vi "S8300E_SetRTCTime_FromSFCS.vi"() -> ()   [LabVIEW 2011]
uses:
  Instance           3 34Saved   MojoMP_SetRTCTime_FromSFCS .vi
  Instance           5 34Saved   MojoMP_SetRTCTime_FromSFCS .vi
  Instance           6 34Saved   MojoMP_SetRTCTime_FromSFCS .vi
  data/MCSDLL.dll
panel:
  out "UUT Msg":string
  out "SFCS Msg":string
  out "VISA resource name out":refnum<visa-resource-name>
  out "begin time":u32
  out "toS8300E_RTC_Data":string
  out "SFCS_Time":string
  out "SFCS_DATE_STRING":string
  out "output param":string
  out "STAGE":string
  out "SFCS_IP":string
  in  "URL":string
  # "設定標準時間\nSetRTC Time from SFCS To S8300E"
  # "2014-9-3"
  # "Error Code:RTC\nError Code:UART"
  # "COM9"
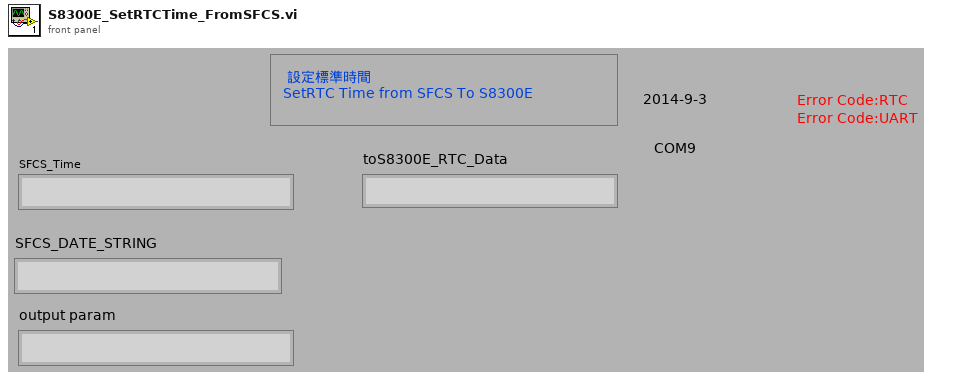
[diagram p1: front panel]
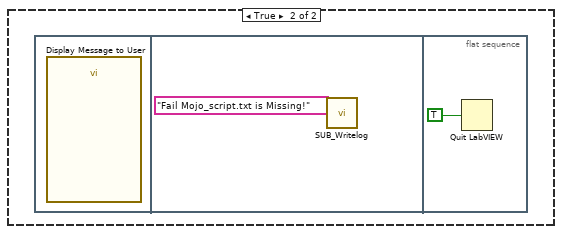
[diagram p3: hidden frame]
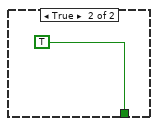
[diagram p9: hidden frame]
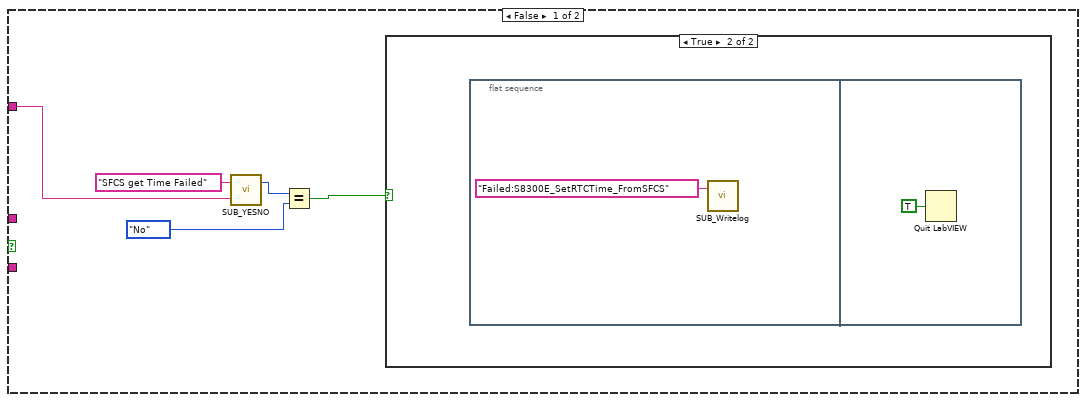
[diagram p10: hidden frame]
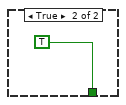
[diagram p13: hidden frame]
diagram:
  n1 = flat-sequence {
    tunnel: [w4] -> w1
    tunnel: w1 -> [w27]
    frame #0 {
      n2 = Tick Count (ms)() -> (millisecond timer value=→"begin time":u32)
    }
    frame #1 {
      n3 = call "SUB_Read_specifFile.vi"("name or relative path"="S8300E_sfcs_misc.txt" ("Script FileName")) -> ("error out"=w7:errorcluster, "text"=w4:string)  [unwired: 1 in]
      n4 = Unbundle By Name(w7) -> ("code"=w6:i32)
      n5 = Not Equal To 0?(x=w6) -> (x != 0?=w5:bool)
      n6 = case shown="False" w5 {
        tunnel: w4 -> [w8 _]
        frame False {
          n7 = flat-sequence {
            tunnel: w8 -> [w14]
            frame #0 {
              n8 = To Upper Case(1:"SFCS_IP=" ("string")) -> (0:w18:string)
              n9 = To Upper Case(1:w14) -> (0:w19:string)
              n10 = call <vilib>:"Trim Whitespace.vi"("string"=w18) -> ("trimmed string"=w16:string)  [unwired: 1 in]
              n11 = call <vilib>:"Trim Whitespace.vi"("string"=w19) -> ("trimmed string"=w15:string)  [unwired: 1 in]
              n12 = Match Pattern(string=w15, regular expression=w16) -> (after substring=w13:string)  [unwired: 1 in, 3 out]
              n13 = Match Pattern(string=w13, regular expression=";") -> (before substring=w11:string)  [unwired: 1 in, 3 out]
              "SFCS_IP" <- w11
              n14 = Equal?(x=w11, y="") -> (x = y?=w9:bool)
              n15 = case shown="True" w9 {
                frame False {
                }
                frame True {
                  n16 = flat-sequence {
                    frame #0 {
                      n17 = call "Display Message to User2"() -> ()  [unwired: 10 in, 2 out]
                    }
                    frame #1 {
                      n18 = call "SUB_Writelog.vi"("Pass/Fail"="Fail Not Found SFCS_IP=\"xx.xx.xx.xx\" in Mojo_script.txt !") -> ()  [unwired: 2 in]
                    }
                    frame #2 {
                      n19 = Quit LabVIEW(quit? (T)=TRUE) -> ()
                    }
                  }
                }
              }
            }
          }
        }
        frame True {
          n20 = flat-sequence {
            frame #0 {
              n21 = call "Display Message to User"() -> ()  [unwired: 10 in, 2 out]
            }
            frame #1 {
              n22 = call "SUB_Writelog.vi"("Pass/Fail"="Fail Mojo_script.txt is Missing!") -> ()  [unwired: 2 in]
            }
            frame #2 {
              n23 = Quit LabVIEW(quit? (T)=TRUE) -> ()
            }
          }
        }
      }
    }
    frame #2 {
      n24 = To Upper Case(1:"SFCS_STAGE=" ("string")) -> (0:w33:string)
      n25 = To Upper Case(1:w27) -> (0:w34:string)
      n26 = call <vilib>:"Trim Whitespace.vi"("string"=w33) -> ("trimmed string"=w32:string)  [unwired: 1 in]
      n27 = call <vilib>:"Trim Whitespace.vi"("string"=w34) -> ("trimmed string"=w31:string)  [unwired: 1 in]
      n28 = Match Pattern(string=w31, regular expression=w32) -> (after substring=w30:string)  [unwired: 1 in, 3 out]
      n29 = Match Pattern(string=w30, regular expression=";") -> (before substring=w26:string)  [unwired: 1 in, 3 out]
      "STAGE" <- w26
      n30 = Not Equal?(x=w26, y="") -> (x != y?=w24:bool)
      n31 = case shown="False" w24 {
        frame False {
          n32 = flat-sequence {
            frame #0 {
              n33 = call "Display Message to User4"() -> ()  [unwired: 10 in, 2 out]
            }
            frame #1 {
              n34 = call "SUB_Writelog.vi"("Pass/Fail"="Fail :Stage  not define in script file!") -> ()  [unwired: 2 in]
            }
            frame #2 {
              n35 = Quit LabVIEW(quit? (T)=TRUE) -> ()
            }
          }
        }
        frame True {
        }
      }
    }
    frame #3 {
      n36 = local read "SFCS_IP"() -> (w37:string)
      n37 = local write "URL"(w37) -> ()
    }
    frame #4 {
      n38 = case shown="True" TRUE {
        frame False {
        }
        frame True {
          n39 = call "SUB_COM1_CLOSE.vi"("VISA resource name"=refnum<visa-resource-name> "COM9") -> ()  [unwired: 3 in]
        }
      }
    }
    frame #5 {
      n40 = case shown="True" TRUE {
        frame False {
        }
        frame True {
          n41 = call "SUB_COM9_INIT.vi"("baud rate"=u32 115200) -> ("VISA resource name out"=w44:refnum<visa-resource-name>)  [unwired: 1 in, 1 out]
          "VISA resource name out" <- w44
          n42 = call "SUB_COM1Wrt.vi"("VISA resource name"=w44, "write buffer"="\r") -> ("duplicate VISA resource name"=w41:refnum<visa-resource-name>)  [unwired: 2 out]
          n43 = call "SUB_ContinueCom1Read.vi"("Numeric"=1200, "duplicate VISA resource name 2"=w41) -> ()  [unwired: 1 in, 3 out]
        }
      }
    }
    frame #6 {
      n44 = case shown="True" TRUE {
        frame False {
        }
        frame True {
          n45 = while {
            stop <- w56 stop-if-true
            w49 = "S8300E" ("Find this String")
            w50 = "\r"
            n46 = Tick Count (ms)() -> (millisecond timer value=w53:u32)
            n47 = local read "VISA resource name out"() -> (w55:refnum<visa-resource-name>)
            n48 = Concatenate Strings(w50, w50, w50) -> (w51:string)
            n49 = call "SUB_COM1Wrt.vi"("VISA resource name"=w55, "write buffer"=w51) -> ("duplicate VISA resource name"=w54:refnum<visa-resource-name>)  [unwired: 2 out]
            n50 = call "SUB_READ_COM1_FindString_timeout.vi"("Find this String"=w49, "Timeout Seccond"=3.0, "Begin time"=w53, "duplicate VISA resource name 2"=w54) -> ("Output String"=w48:string)  [unwired: 1 in, 2 out]
            n51 = call "SUB_FindSpecificString.vi"("Find this String"=w49, "String data"=w48) -> ("Found"=w47:bool)  [unwired: 2 in, 1 out]
            n52 = case shown="False" w47 {
              tunnel: w48 -> [w61 _]
              tunnel: [w57 TRUE] -> w56
              frame False {
                n53 = call "SUB_YESNO.vi"("Debug View"=w61, "Status"="UART無正確反應!需有S8300E字串") -> ("yes/no"=w60:enum32{"No Selection", "Yes", "No", "None"})  [unwired: 1 in]
                n54 = Equal?(x=w60, y=enum32{"No Selection", "Yes", "No", "None"}."No") -> (x = y?=w58:bool)
                n55 = case shown="True" w58 {
                  tunnel: [_ w63] -> w57
                  frame False {
                  }
                  frame True {
                    n56 = flat-sequence {
                      tunnel: [w67] -> w63
                      frame #0 {
                        n57 = call "SUB_Writelog.vi"("Pass/Fail"="Fail:S8300E_SetRTCTime_FromSFCS") -> ()  [unwired: 2 in]
                      }
                      frame #1 {
                        n58 = call "SUB_SFCS_SendResult.vi"("ErrorCode"="UART", "PASS_Fail (1/0)"=i8 0) -> ()  [unwired: 1 out]
                      }
                      frame #2 {
                        w67 = TRUE ("quit? (T)")
                        n59 = Quit LabVIEW(quit? (T)=w67) -> ()
                      }
                    }
                  }
                }
              }
              frame True {
              }
            }
          }
        }
      }
    }
    frame #7 {
      n60 = while {
        stop <- w69 stop-if-true
        w86 = ":" ("regular expression")
        w88 = "/" ("regular expression")
        w90 = " " ("regular expression")
        n61 = local read "STAGE"() -> (w94:string)
        n62 = To Upper Case(1:"NG" ("string")) -> (0:w101:string)
        n63 = To Upper Case(1:"Fail" ("string")) -> (0:w78:string)
        n64 = call <vilib>:"Trim Whitespace.vi"("string"=w101) -> ("trimmed string"=w98:string)  [unwired: 1 in]
        n65 = call <vilib>:"Trim Whitespace.vi"("string"=w78) -> ("trimmed string"=w75:string)  [unwired: 1 in]
        n66 = dll-call lib="D:/S8300E_Project/data/MCSDLL.dll" fn="SFCS_GetCurrentDBSysdate"("URL"="URL", "Stage"=w94, "TimeFormat"="YYYY/MM/DD HH24:MI:SS") -> (w70:string)  [unwired: 6 in, 2 out]
        "output param" <- w70
        "SFCS Msg" <- w70
        n67 = To Upper Case(1:w70) -> (0:w102:string)
        n68 = To Upper Case(1:w70) -> (0:w79:string)
        n69 = call <vilib>:"Trim Whitespace.vi"("string"=w102) -> ("trimmed string"=w97:string)  [unwired: 1 in]
        n70 = call <vilib>:"Trim Whitespace.vi"("string"=w79) -> ("trimmed string"=w74:string)  [unwired: 1 in]
        n71 = Match Pattern(string=w97, regular expression=w98) -> (match substring=w99:string)  [unwired: 1 in, 3 out]
        n72 = Match Pattern(string=w74, regular expression=w75) -> (match substring=w76:string)  [unwired: 1 in, 3 out]
        n73 = Not Equal?(x=w99, y=w98) -> (x != y?=w73:bool)
        n74 = Not Equal?(x=w76, y=w75) -> (x != y?=w72:bool)
        n75 = Match Pattern(string=w70, regular expression=w86) -> (match substring=w87:string)  [unwired: 1 in, 3 out]
        n76 = Match Pattern(string=w70, regular expression=w88) -> (match substring=w89:string)  [unwired: 1 in, 3 out]
        n77 = And(x=w73, y=w72) -> (x .and. y?=w71:bool)
        n78 = Equal?(x=w89, y=w88) -> (x = y?=w83:bool)
        n79 = Equal?(x=w87, y=w86) -> (x = y?=w85:bool)
        n80 = Match Pattern(string=w70, regular expression=w90) -> (before substring=w93:string, match substring=w91:string, after substring=w92:string)  [unwired: 1 in, 1 out]
        n81 = And(x=w85, y=w71) -> (x .and. y?=w81:bool)
        n82 = Equal?(x=w91, y=w90) -> (x = y?=w84:bool)
        n83 = And(x=w84, y=w83) -> (x .and. y?=w82:bool)
        n84 = And(x=w82, y=w81) -> (x .and. y?=w80:bool)
        n85 = case shown="True" w80 {
          tunnel: w93 -> [_ w115]
          tunnel: w92 -> [_ w114]
          tunnel: w70 -> [w103 _]
          tunnel: [_ w113] -> w69
          frame False {
            n86 = call "SUB_YESNO.vi"("Debug View"=w103, "Status"="SFCS get Time Failed") -> ("yes/no"=w106:enum32{"No Selection", "Yes", "No", "None"})  [unwired: 1 in]
            n87 = Equal?(x=w106, y=enum32{"No Selection", "Yes", "No", "None"}."No") -> (x = y?=w104:bool)
            n88 = case shown="True" w104 {
              frame False {
              }
              frame True {
                n89 = flat-sequence {
                  frame #0 {
                    n90 = call "SUB_Writelog.vi"("Pass/Fail"="Failed:S8300E_SetRTCTime_FromSFCS") -> ()  [unwired: 2 in]
                  }
                  frame #1 {
                    n91 = Quit LabVIEW(quit? (T)=TRUE) -> ()
                  }
                }
              }
            }
          }
          frame True {
            n92 = flat-sequence {
              tunnel: w115 -> [w131]
              tunnel: w114 -> [w130]
              tunnel: [w117] -> w112
              tunnel: w112 -> [w133]
              tunnel: [w132] -> w110
              tunnel: [w137] -> w111
              tunnel: w110 -> [w137]
              tunnel: [w145] -> w113
              tunnel: w111 -> [w139]
              frame #0 {
                n93 = call <vilib>:"Trim Whitespace.vi"("string"=w131) -> ("trimmed string"=w122:string)  [unwired: 1 in]
                "SFCS_DATE_STRING" <- w122
                n94 = call <vilib>:"Trim Whitespace.vi"("string"=w130) -> ("trimmed string"=w129:string)  [unwired: 1 in]
                "SFCS_Time" <- w129
                n95 = call "SUB_OUT_THIS_token.vi"("Remove token symbl1 3"="", "Remove token symbl1 2"=":" ("Remove token symbl1"), "Remove token symbl1"="/", "input string"=w129) -> ("result string"=w120:string)  [unwired: 1 in]
                n96 = call "SUB_OUT_THIS_token.vi"("Remove token symbl1 3"="", "Remove token symbl1 2"=":" ("Remove token symbl1"), "Remove token symbl1"="/", "input string"=w122) -> ("result string"=w121:string)  [unwired: 1 in]
                n97 = Concatenate Strings(w121, w120) -> (w116:string)
                "toS8300E_RTC_Data" <- w116
                n98 = Concatenate Strings("./rtc.sh -w  ", w116, "\r") -> (w117:string)
              }
              frame #1 {
                n99 = local read "VISA resource name out"() -> (w135:refnum<visa-resource-name>)
                n100 = call "SUB_ContinueCom1Read.vi"("Numeric"=1200, "duplicate VISA resource name 2"=w135) -> ("duplicate VISA resource name"=w134:refnum<visa-resource-name>)  [unwired: 1 in, 2 out]
                n101 = call "SUB_COM1Wrt.vi"("VISA resource name"=w134, "write buffer"=w133) -> ("duplicate VISA resource name"=w132:refnum<visa-resource-name>)  [unwired: 2 out]
              }
              frame #2 {
                n102 = Wait (ms)(milliseconds to wait=u32 3000) -> ()  [unwired: 1 out]
              }
              frame #3 {
                n103 = Tick Count (ms)() -> (millisecond timer value=w141:u32)
                n104 = call "SUB_READ_COM1_FindString_timeout.vi"("Find this String"="PASSED=", "Timeout Seccond"=1.0, "Begin time"=w141, "duplicate VISA resource name 2"=w139) -> ("Output String"=→"UUT Msg":string, "Found String"=w143:bool)  [unwired: 1 in, 1 out]
                n105 = case shown="False" w143 {
                  tunnel: [_ TRUE] -> w145
                  frame False {
                    n106 = local read "UUT Msg"() -> (w149:string)
                    n107 = call "SUB_YESNO.vi"("Debug View"=w149, "Status"="設定RTC失敗!") -> ("yes/no"=w148:enum32{"No Selection", "Yes", "No", "None"})  [unwired: 1 in]
                    n108 = Equal?(x=w148, y=enum32{"No Selection", "Yes", "No", "None"}."No") -> (x = y?=w146:bool)
                    n109 = case shown="True" w146 {
                      frame False {
                      }
                      frame True {
                        n110 = flat-sequence {
                          frame #0 {
                            n111 = call "SUB_SFCS_SendResult.vi"("ErrorCode"="RTC", "PASS_Fail (1/0)"=i8 0) -> ()  [unwired: 1 out]
                          }
                          frame #1 {
                            n112 = call "SUB_Writelog.vi"("Pass/Fail"="Failed:S8300E_SetRTCTime_FromSFCS") -> ()  [unwired: 2 in]
                          }
                          frame #2 {
                            n113 = Quit LabVIEW(quit? (T)=TRUE) -> ()
                          }
                        }
                      }
                    }
                  }
                  frame True {
                  }
                }
              }
            }
          }
        }
      }
    }
    frame #8 {
      n114 = local read "VISA resource name out"() -> (w156:refnum<visa-resource-name>)
      n115 = call "SUB_COM1_CLOSE.vi"("VISA resource name"=w156) -> ()  [unwired: 3 in]
    }
    frame #9 {
      w159 = "\r"
      n116 = local read "SFCS Msg"() -> (w162:string)
      n117 = local read "UUT Msg"() -> (w160:string)
      n118 = Tick Count (ms)() -> (millisecond timer value=w166:u32)
      n119 = local read "begin time"() -> (w167:u32)
      n120 = call "SUB_CAL_TESTTIME.vi"("Test Item name"="S8300E_SetRTCTime_FromSFCS", "Stop tick time"=w166, "Start tick time"=w167) -> ("Test Time output"=w158:string)  [unwired: 2 in]
      n121 = Concatenate Strings("Pass :S8300E_SetRTCTime_FromSFCS" ("Pass/Fail"), w159, "SFCS Message:", w162, w159, "UUT Message:", w160, w159, w158) -> (w157:string)
      n122 = call "SUB_Writelog.vi"("Pass/Fail"=w157) -> ()  [unwired: 2 in]
    }
    frame #10 {
      n123 = Quit LabVIEW(quit? (T)=TRUE) -> ()
    }
  }
